vi "gfitsio-allocate-memory-for-image-read.vi"() -> (1 "Numeric 3":i32, 2 "Numeric 2":i32, 3 "Numeric":i32)   [LabVIEW 2011, in "gfitsio.lvlib"]
uses:
  gfitsio.lvlib
panel:
  in  "inc":i32[](array[numeric])
  in  "lpixel":i32[](array[numeric])
  in  "fpixel":i32[](array[numeric])
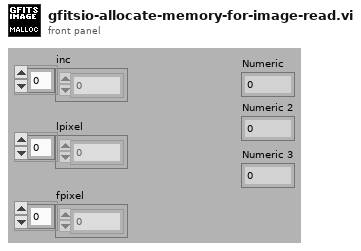
[diagram p1: front panel]
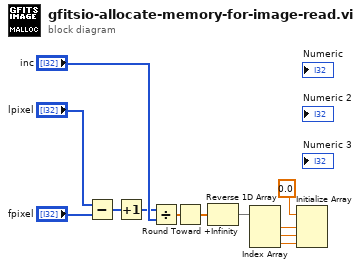
[diagram p0: block diagram]
diagram:
  n1 = Subtract(x="lpixel", y="fpixel") -> (x-y=w6:i32[])
  n2 = Increment(x=w6) -> (x+1=w7:i32[])
  n3 = Divide(x=w7, y="inc") -> (x/y=w3:dbl[])
  n4 = Round Toward +Infinity(x=w3) -> (ceil(x): smallest int >= x=w9:dbl[])
  n5 = Reverse 1D Array(array=w9) -> (reversed array=w8:dbl[])
  n6 = Index Array(array=w8) -> (element #1=w4:dbl, element #2=w5:dbl, element #3=w10:dbl)  [unwired: 3 in]
  n7 = Initialize Array(sgl 0.0, w4, w5, w10) -> (w2:sgl[][][])
